vi "Read Value.vi"(7 "AnalogIn":refnum<class "AI.lvclass">, 8 "error in (no error)":errorcluster, 11 "Session In":refnum<class "Session.lvclass">) -> (0 "error out":errorcluster, 2 "Value":T1, 3 "Session Out":refnum<class "Session.lvclass">)   [LabVIEW 2024, in "CTI.lvlib" / "AI.lvclass"]
uses:
  AI.lvclass
  Session/Session.lvclass
  Raw ADC.ctl
  AI.lvclass/AI.ctl
  CTI.lvlib
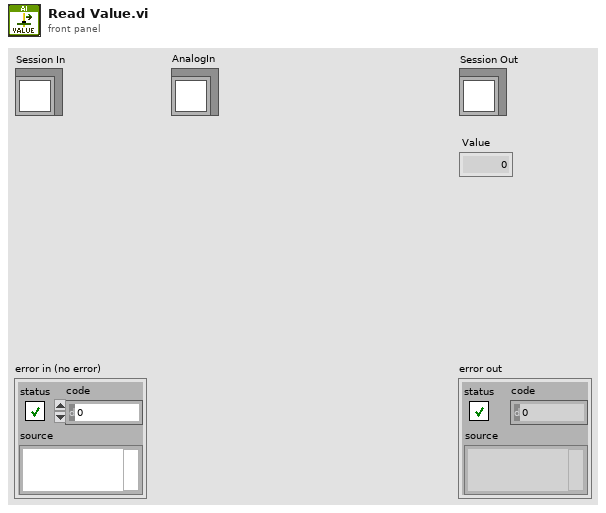
[diagram p1: front panel]
types:
  T1 = typedef "CTI.lvlib/Raw ADC.ctl" = u16
  T2 = typedef "CTI.lvlib/ADC Number.ctl" = i8
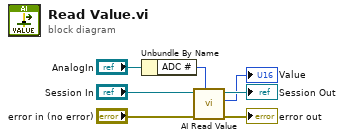
[diagram p0: block diagram]
diagram:
  n1 = Unbundle By Name("AnalogIn") -> ("ADC #"=w1:T2)
  n2 = call "AI Read Value.vi"("ADC #"=w1, "error in (no error)"="error in (no error)", "Session in"="Session In") -> ("error out"=→"error out":errorcluster, "Value"=→"Value":T1, "Session out"=→"Session Out":refnum<class "Session.lvclass">)  [unwired: 6 in]
